vi "Tipping Device Test.vi"(10 "Progress":string, 11 "ProgressText":string) -> (3 "EndTestText":string)   [LabVIEW 2012]
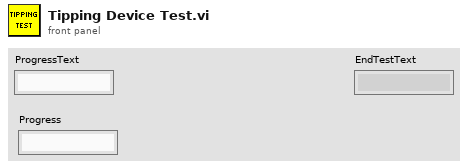
[diagram p1: front panel]
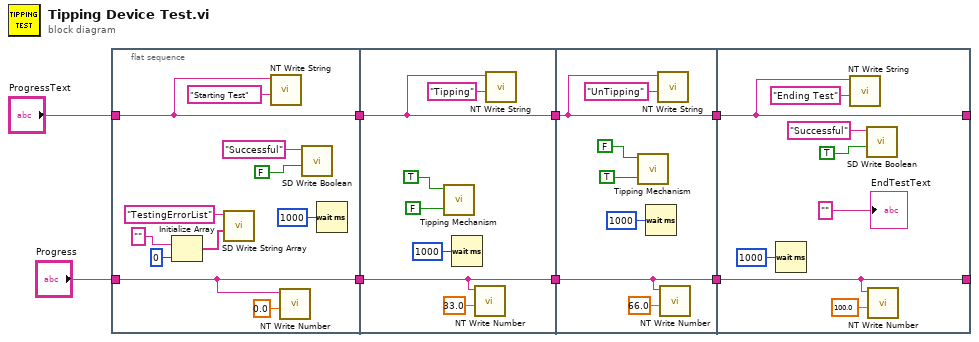
[diagram p0: block diagram]
diagram:
  n1 = flat-sequence {
    tunnel: [w11] -> w8
    tunnel: "ProgressText" -> [w11]
    tunnel: [w10] -> w6
    tunnel: "Progress" -> [w10]
    tunnel: w8 -> [w25]
    tunnel: w6 -> [w22]
    tunnel: [w25] -> w4
    tunnel: [w22] -> w3
    tunnel: w4 -> [w32]
    tunnel: w3 -> [w28]
    tunnel: [w32] -> w2
    tunnel: [w28] -> w1
    tunnel: w2 -> [w40]
    tunnel: w1 -> [w36]
    tunnel: [w40] -> _
    tunnel: [w36] -> _
    frame #0 {
      n2 = Initialize Array("", 0 ("dimension size")) -> (w14:string[])
      n3 = call <vilib>:"SD Write String Array.vi"("String Array"=w14, "Name"="TestingErrorList") -> ()  [unwired: 8 in, 2 out]
      n4 = call <vilib>:"NT Write String.vi"("String"="Starting Test", "Name"=w11) -> ()  [unwired: 9 in, 1 out]
      n5 = call <vilib>:"NT Write Number.vi"("Numeric"=0.0, "Name"=w10) -> ()  [unwired: 9 in, 1 out]
      n6 = call <vilib>:"SD Write Boolean.vi"("Boolean"=FALSE, "Name"="Successful") -> ()  [unwired: 8 in, 2 out]
      n7 = Wait (ms)(milliseconds to wait=u32 1000) -> ()  [unwired: 1 out]
    }
    frame #1 {
      n8 = call "Tipping Mechanism.vi"("Un-Tip"=FALSE, "Tip"=TRUE) -> ()  [unwired: 10 in]
      n9 = Wait (ms)(milliseconds to wait=u32 1000) -> ()  [unwired: 1 out]
      n10 = call <vilib>:"NT Write Number.vi"("Numeric"=33.0, "Name"=w22) -> ()  [unwired: 9 in, 1 out]
      n11 = call <vilib>:"NT Write String.vi"("String"="Tipping", "Name"=w25) -> ()  [unwired: 9 in, 1 out]
    }
    frame #2 {
      n12 = call "Tipping Mechanism.vi"("Un-Tip"=TRUE, "Tip"=FALSE) -> ()  [unwired: 10 in]
      n13 = Wait (ms)(milliseconds to wait=u32 1000) -> ()  [unwired: 1 out]
      n14 = call <vilib>:"NT Write String.vi"("String"="UnTipping", "Name"=w32) -> ()  [unwired: 9 in, 1 out]
      n15 = call <vilib>:"NT Write Number.vi"("Numeric"=66.0, "Name"=w28) -> ()  [unwired: 9 in, 1 out]
    }
    frame #3 {
      n16 = Wait (ms)(milliseconds to wait=u32 1000) -> ()  [unwired: 1 out]
      n17 = call <vilib>:"NT Write String.vi"("String"="Ending Test", "Name"=w40) -> ()  [unwired: 9 in, 1 out]
      n18 = call <vilib>:"SD Write Boolean.vi"("Boolean"=TRUE, "Name"="Successful") -> ()  [unwired: 8 in, 2 out]
      n19 = call <vilib>:"NT Write Number.vi"("Numeric"=100.0, "Name"=w36) -> ()  [unwired: 9 in, 1 out]
      "EndTestText" <- "" ("EndTestText")
    }
  }
